vi "JointsAngle2XY.vi"(9 "Corrected joint 2":dbl, 10 "Corrected joint 1":dbl) -> (1 "y":dbl, 2 "x":dbl)   [LabVIEW 2023]
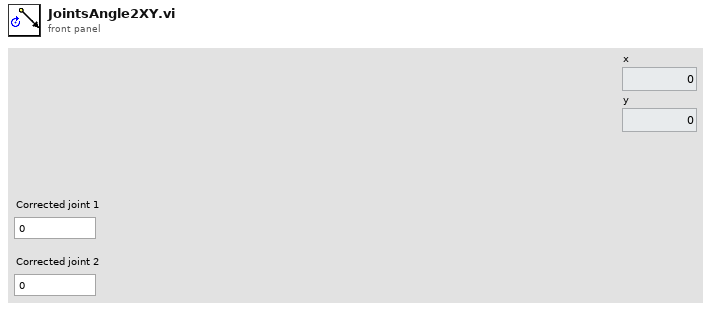
[diagram p1: front panel]
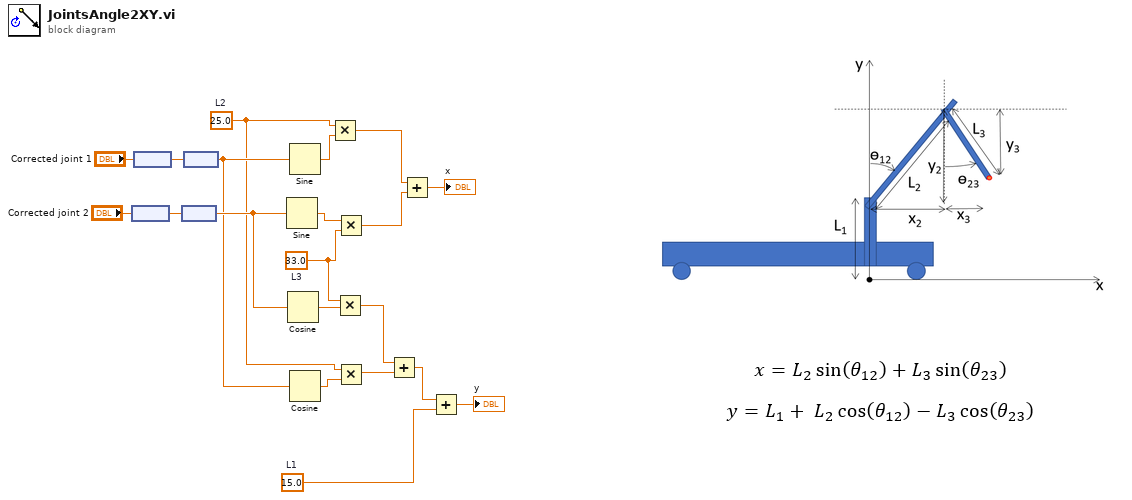
[diagram p0: block diagram]
diagram:
  w2 = 25.0  # L2
  w8 = 33.0  # L3
  w11 = 15.0  # L1
  n1 = node("Corrected joint 2") -> (w17:dbl[unit])
  n2 = node("Corrected joint 1") -> (w19:dbl[unit])
  n3 = node(w17) -> (w10:dbl)
  n4 = node(w19) -> (w5:dbl)
  n5 = Sine(x=w10) -> (sin(x)=w15:dbl)
  n6 = Cosine(x=w10) -> (cos(x)=w9:dbl)
  n7 = Sine(x=w5) -> (sin(x)=w20:dbl)
  n8 = Cosine(x=w5) -> (cos(x)=w4:dbl)
  n9 = Multiply(x=w2, y=w20) -> (x*y=w14:dbl)
  n10 = Multiply(x=w8, y=w9) -> (x*y=w6:dbl)
  n11 = Multiply(x=w15, y=w8) -> (x*y=w13:dbl)
  n12 = Multiply(x=w2, y=w4) -> (x*y=w3:dbl)
  n13 = Add(x=w6, y=w3) -> (x+y=w7:dbl)
  n14 = Add(x=w14, y=w13) -> (x+y=→"x":dbl)
  n15 = Add(x=w7, y=w11) -> (x+y=→"y":dbl)
